vi "Get Control References By Match Pattern.vi"(4 "error in (no error)":errorcluster, 5 "regular expression":string, 7 "Control references":cluster{string, refnum<vi>}[](array[cluster])) -> (0 "error out":errorcluster, 2 "References":refnum<vi>[](array[refnum]))   [LabVIEW 2014]
doc: "This VI will give you a 1D array of control refrences by feeding it the output of the\" get reference to all controls\" VI and a Match Pattern regex to match the names for the controls you would like a reference to."
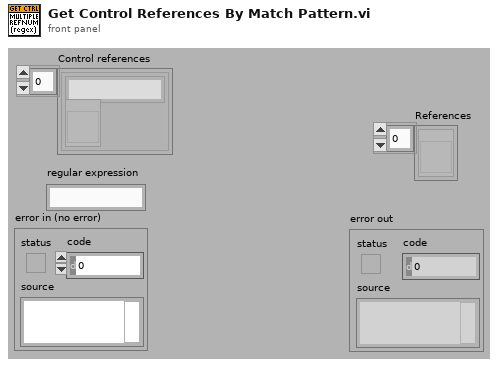
[diagram p1: front panel]
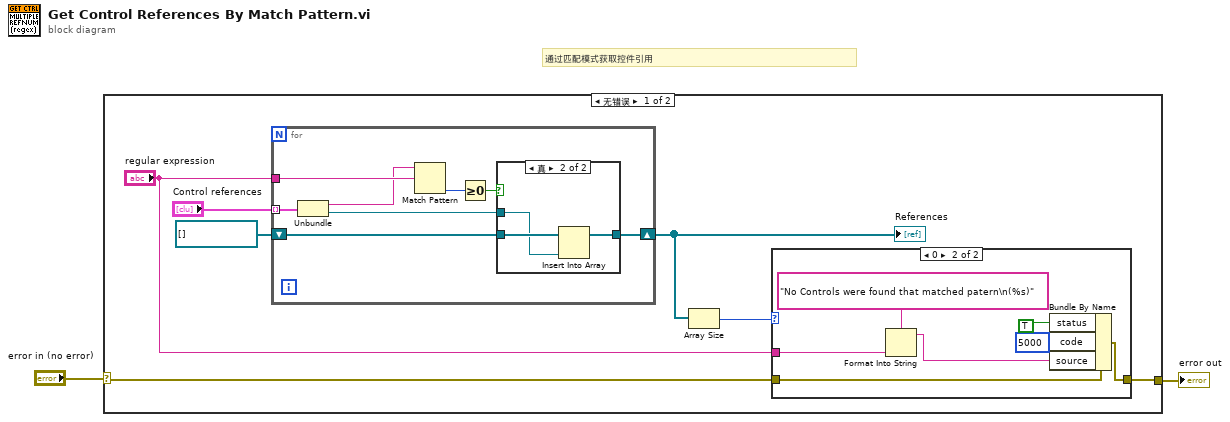
[diagram p0: block diagram]
diagram:
  # "通过匹配模式获取控件引用"
  n1 = case shown="无错误" "error in (no error)" {
    selector: "error in (no error)" -> [w5 w30]
    tunnel: [w4 w30] -> w2
    frame No Error {
      n2 = for {
        tunnel: "regular expression" -> [w25]
        tunnel: "Control references" -> [w24] mode=indexing
        shift-right: [w20] -> w7
        shift-left: refnum<vi>[] [] -> [w18]
        n3 = Unbundle(w24) -> (w23:string, w19:refnum<vi>)
        n4 = Match Pattern(string=w23, regular expression=w25) -> (offset past match=w22:i32)  [unwired: 1 in, 3 out]
        n5 = Greater Or Equal To 0?(x=w22) -> (x >= 0?=w21:bool)
        n6 = case shown="真" w21 {
          tunnel: [w26 w28] -> w20
          tunnel: w19 -> [_ w27]
          tunnel: w18 -> [w26 w29]
          frame False {
          }
          frame True {
            n7 = Insert Into Array(array=w29, new element=w27) -> (w28:refnum<vi>[])  [unwired: 1 in]
          }
        }
      }
      "References" <- w7
      n8 = Array Size(array=w7) -> (size(s)=w8:i32)
      n9 = case shown="0" w8 {
        tunnel: w5 -> [w10 w14]
        tunnel: [w10 w13] -> w4
        tunnel: "regular expression" -> [_ w11]
        frame Default {
        }
        frame 0 {
          n10 = Format Into String(format string="No Controls were found that matched patern\n(%s)", w11) -> (resulting string=w17:string)  [unwired: 2 in, 1 out]
          n11 = Bundle By Name(cluster=w14, "status"=TRUE ("Error/Warning"), "code"=5000, "source"=w17) -> (w13:errorcluster)
        }
      }
    }
    frame Error {
    }
  }
  "error out" <- w2
